vi "WASh controller.vi"(8 "error in (no error)":errorcluster) -> (0 "error out":errorcluster)   [LabVIEW 2015]
doc: "Controller performs all mathematical and logical operations of the application. It is an independent module which communicates with othe modules sending and receiving messaging."
uses:
  type defs/WASH controller states.ctl
  type defs/WASH communication module tasks.ctl
  type defs/WASH step selection buttons.ctl
  type defs/WASH indicators.ctl
  type defs/WASH error levels.ctl
  type defs/WASH simulated database tasks.ctl
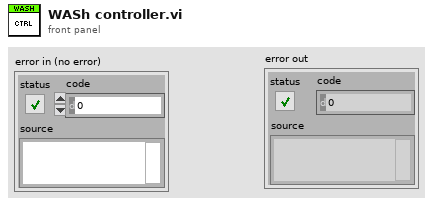
[diagram p1: front panel]
types:
  T1 = typedef "WASH controller states.ctl" = enum16{"initialize", "wait for start", "start", "wait for vehicle position", "wash step execute", "wash step complete", "wash exit", "wash abort"}
  T2 = typedef "WASH error levels.ctl" = enum16{"minor", "wash cycle", "system"}
  T3 = typedef "WASH communication module tasks.ctl" = enum16{"init", "enable controls", "update wash indicators", "update wash entry", "update vehicle out of pos", "update timing", "set step buttons values", "set start button value", "set vehicle position entry", "wait for input", "close"}
  T4 = typedef "WASH simulated database tasks.ctl" = enum16{"init", "read", "insert record", "update record", "query timing", "close"}
  T5 = typedef "WASH indicators.ctl" = cluster{"Under body wash":bool, "bug remover":bool, "Pre-soak":bool, "High pressure wash":bool, "Low pressure wax":bool, "Spot free rinse":bool, "Tire shine foam":bool, "Air dry":bool}
  T6 = typedef "WASH step selection buttons.ctl" = cluster{"Under body wash":bool, "Bug remover":bool, "Pre-soak":bool, "High pressure wash":bool, "Low pressure wax":bool, "Spot free rinse":bool, "Tire shine foam":bool, "Air dry":bool}
  T7 = enum8{"Enabled", "Disabled", "Disabled and Grayed Out"}
  T8 = typedef "WASH UI to CTRL commands.ctl" = enum16{"start button pushed", "vehicle position changed"}
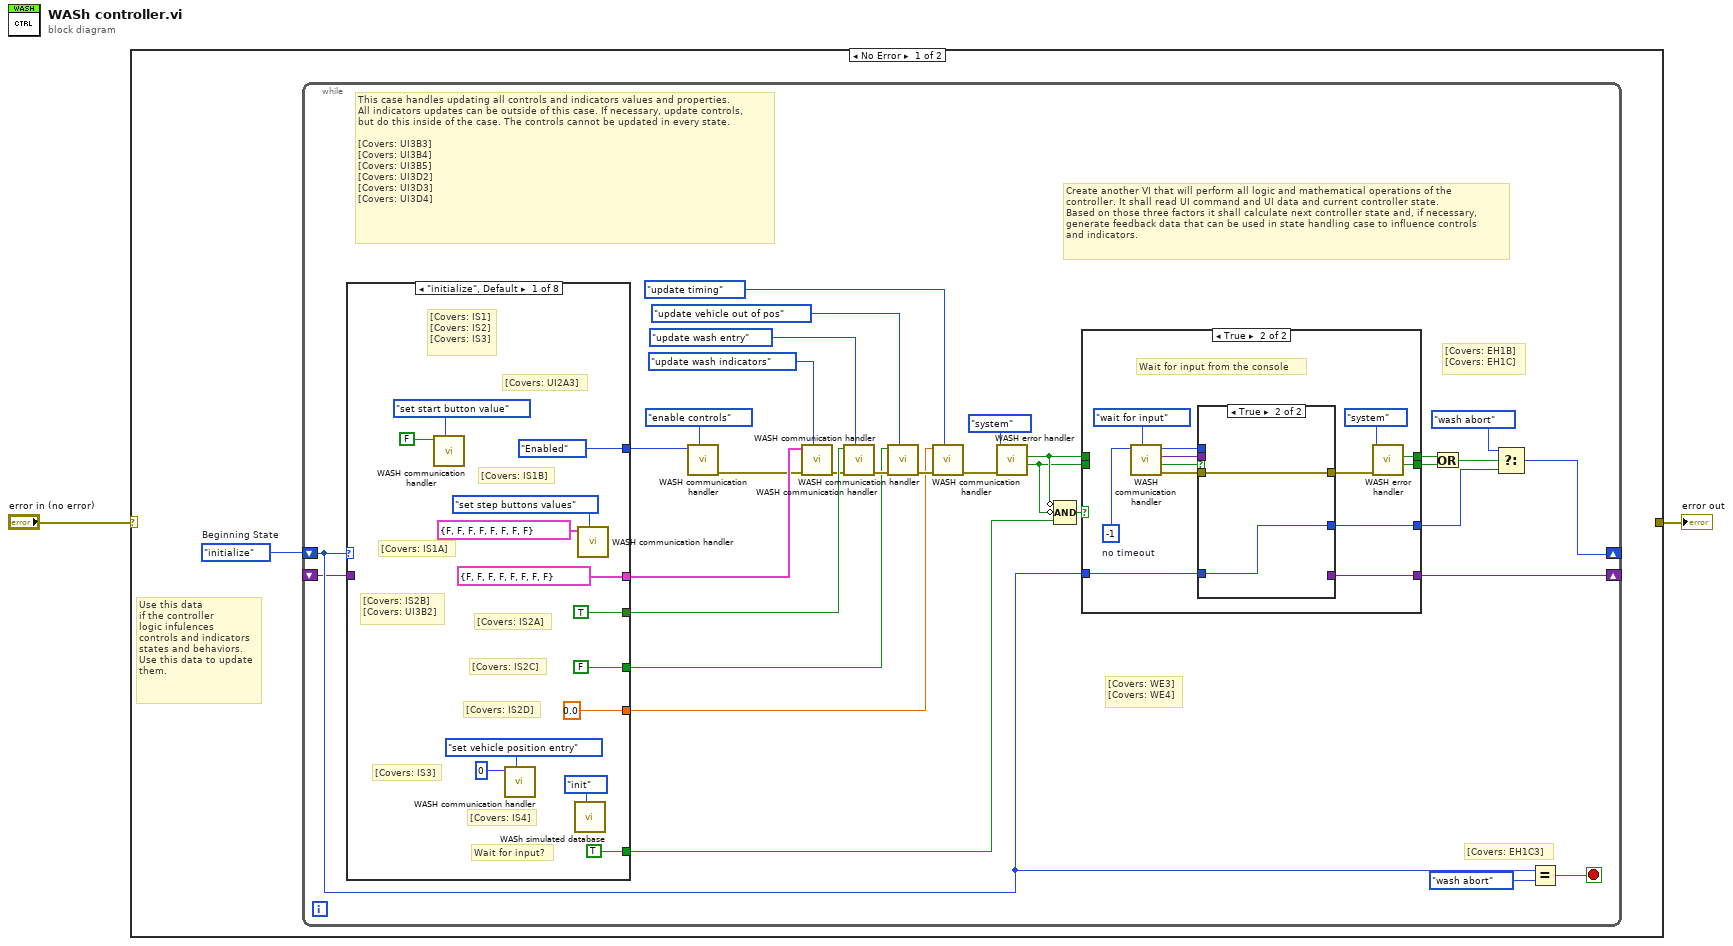
[diagram p0: block diagram]
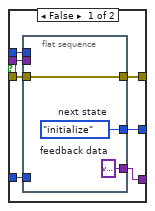
[diagram p3: hidden frame]
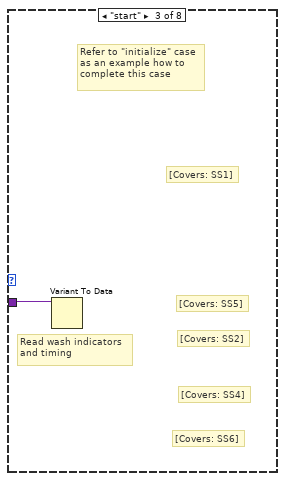
[diagram p5: hidden frame]
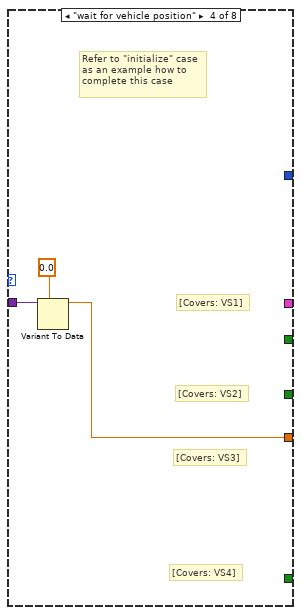
[diagram p6: hidden frame]
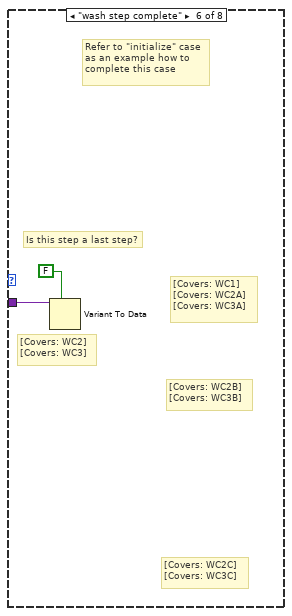
[diagram p8: hidden frame]
diagram:
  n1 = case shown="No Error" "error in (no error)" {
    selector: "error in (no error)" -> [_ w82]
    tunnel: [_ w82] -> w1
    frame No Error {
      w3 = WASH_controller_states."initialize"  # Beginning State
      # "Use this data\nif the controller\nlogic infulences\ncontrols and indicators\nstates and behaviors.\nUse this data to update\nthem."
      n2 = while {
        shift-right: [w9] -> _
        shift-left: w3 -> [w8]
        shift-right: [w4] -> _
        shift-left: _ -> [w5]
        stop <- w7 stop-if-true
        # "[Covers: WE3]\n[Covers: WE4]"
        # "Create another VI that will perform all logic and mathematical operations of the\ncontroller. It shall read UI command and UI data and current controller state.\nBased on those three factors it shall calculate next controller state and, if necessary,\ngenerate feedback data that can be used in state handling case to influence controls\nand indicators."
        # "[Covers: EH1C3]"
        # "[Covers: EH1B]\n[Covers: EH1C]"
        # "This case handles updating all controls and indicators values and properties.\nAll indicators updates can be outside of this case. If necessary, update controls,\nbut do this inside of the case. The controls cannot be updated in every state.\n\n[Covers: UI3B3]\n[Covers: UI3B4]\n[Covers: UI3B5]\n[Covers: UI3D2]\n[Covers: UI3D3]\n[Covers: UI3D4]"
        n3 = case shown="\"initialize\", Default" w8 {
          tunnel: [T7."Enabled" ("Disabled") _ _ _ _ _ _ _] -> w33
          tunnel: [T5 {"Under body wash"=FALSE, "bug remover"=FALSE, "Pre-soak"=FALSE, "High pressure wash"=FALSE, "Low pressure wax"=FALSE, "Spot free rinse"=FALSE, "Tire shine foam"=FALSE, "Air dry"=FALSE} ("wash indicators") _ _ _ _ _ _ _] -> w31
          tunnel: [TRUE _ _ _ _ _ _ _] -> w29
          tunnel: [FALSE _ _ _ _ _ _ _] -> w25
          tunnel: [0.0 _ _ w77 _ _ _ _] -> w21
          tunnel: [TRUE _ _ _ _ _ _ _] -> w15
          tunnel: w5 -> [_ _ w76 w79 _ w81 _ _]
          frame "initialize", Default {
            # "[Covers: UI2A3]"
            # "Wait for input?"
            # "[Covers: IS4]"
            # "[Covers: IS3]"
            # "[Covers: IS2D]"
            # "[Covers: IS2C]"
            # "[Covers: IS1]\n[Covers: IS2]\n[Covers: IS3]"
            # "[Covers: IS2A]"
            # "[Covers: IS2B]\n[Covers: UI3B2]"
            # "[Covers: IS1B]"
            # "[Covers: IS1A]"
            n4 = call "WASH communication handler.vi"("task"=WASH_communication_module_tasks."set start button value", "parameters"=FALSE) -> ()  [unwired: 6 in, 4 out]
            n5 = call "WASH communication handler.vi"("task"=WASH_communication_module_tasks."set vehicle position entry", "parameters"=0) -> ()  [unwired: 6 in, 4 out]
            n6 = call "WASh simulated database.vi"("task"=WASH_simulated_database_tasks."init") -> ()  [unwired: 8 in, 3 out]
            n7 = call "WASH communication handler.vi"("task"=WASH_communication_module_tasks."set step buttons values", "parameters"=T6 {"Under body wash"=FALSE, "Bug remover"=FALSE, "Pre-soak"=FALSE, "High pressure wash"=FALSE, "Low pressure wax"=FALSE, "Spot free rinse"=FALSE, "Tire shine foam"=FALSE, "Air dry"=FALSE} ("Wash step selection")) -> ()  [unwired: 6 in, 4 out]
          }
          frame "wait for start" {
            # "[Covers: WS3]"
            # "[Covers: WS2]"
            # "[Covers: WS1]"
            # "Refer to \"initialize\" case\nas an example how to\ncomplete this case"
          }
          frame "start" {
            # "Read wash indicators\nand timing"
            # "[Covers: SS6]"
            # "[Covers: SS5]"
            # "[Covers: SS4]"
            # "[Covers: SS2]"
            # "Refer to \"initialize\" case\nas an example how to\ncomplete this case"
            # "[Covers: SS1]"
            n8 = Variant To Data(Variant=w76) -> ()  [unwired: 2 in, 2 out]
          }
          frame "wait for vehicle position" {
            # "[Covers: VS4]"
            # "[Covers: VS3]"
            # "[Covers: VS2]"
            # "Refer to \"initialize\" case\nas an example how to\ncomplete this case"
            # "[Covers: VS1]"
            n9 = Variant To Data(type=0.0, Variant=w79) -> (data=w77:dbl)  [unwired: 1 in, 1 out]
          }
          frame "wash step execute" {
            # "[Covers: WX4]"
            # "[Covers: WX3]"
            # "[Covers: WX1]"
            # "[Covers: WX2]"
            # "Refer to \"initialize\" case\nas an example how to\ncomplete this case"
          }
          frame "wash step complete" {
            # "[Covers: WC2C]\n[Covers: WC3C]"
            # "[Covers: WC2B]\n[Covers: WC3B]"
            # "[Covers: WC2]\n[Covers: WC3]"
            # "Is this step a last step?"
            # "Refer to \"initialize\" case\nas an example how to\ncomplete this case"
            # "[Covers: WC1]\n[Covers: WC2A]\n[Covers: WC3A]"
            n10 = Variant To Data(type=FALSE, Variant=w81) -> ()  [unwired: 1 in, 2 out]
          }
          frame "wash exit" {
            # "[Covers: WE2]"
            # "[Covers: WE1]"
            # "Refer to \"initialize\" case\nas an example how to\ncomplete this case"
          }
          frame "wash abort" {
            # "[Covers: TS2]"
            # "[Covers: TS5]"
            # "[Covers: TS4]"
            # "[Covers: TS3]"
            # "[Covers: TS1]"
            # "Refer to \"initialize\" case\nas an example how to\ncomplete this case"
          }
        }
        n11 = call "WASH communication handler.vi"("task"=WASH_communication_module_tasks."enable controls", "parameters"=w33) -> ("error out"=w24:errorcluster)  [unwired: 6 in, 3 out]
        n12 = call "WASH communication handler.vi"("task"=WASH_communication_module_tasks."update wash indicators", "error in (no error)"=w24, "parameters"=w31) -> ("error out"=w28:errorcluster)  [unwired: 5 in, 3 out]
        n13 = call "WASH communication handler.vi"("task"=WASH_communication_module_tasks."update wash entry", "error in (no error)"=w28, "parameters"=w29) -> ("error out"=w27:errorcluster)  [unwired: 5 in, 3 out]
        n14 = call "WASH communication handler.vi"("task"=WASH_communication_module_tasks."update vehicle out of pos", "error in (no error)"=w27, "parameters"=w25) -> ("error out"=w23:errorcluster)  [unwired: 5 in, 3 out]
        n15 = call "WASH communication handler.vi"("task"=WASH_communication_module_tasks."update timing", "error in (no error)"=w23, "parameters"=w21) -> ("error out"=w20:errorcluster)  [unwired: 5 in, 3 out]
        n16 = call "WASH error handler.vi"("error in (no error)"=w20, "error levels"=WASH_error_levels."system") -> ("system error?"=w16:bool, "wash cycle error?"=w17:bool)  [unwired: 7 in, 1 out]
        n17 = Compound Arithmetic op=AND(invert w17, invert w16, w15) -> (w18:bool)
        n18 = case shown="True" w18 {
          tunnel: [w36 w43] -> w12
          tunnel: [w37 w42] -> w10
          tunnel: w17 -> [w37 _]
          tunnel: w16 -> [w36 _]
          tunnel: w8 -> [w35 w40]
          tunnel: [w35 w39] -> w14
          tunnel: [_ w38] -> w4
          frame False {
          }
          frame True {
            w41 = -1  # no timeout
            # "Wait for input from the console"
            n19 = call "WASH communication handler.vi"("task"=WASH_communication_module_tasks."wait for input", "parameters"=w41) -> ("error out"=w48:errorcluster, "timed out?"=w49:bool, "UI data"=w47:variant, "UI command"=w46:T8)  [unwired: 6 in]
            n20 = case shown="True" w49 {
              tunnel: w48 -> [w57 w62]
              tunnel: w47 -> [w54 _]
              tunnel: w46 -> [w53 _]
              tunnel: [w56 w62] -> w45
              tunnel: w40 -> [w55 w61]
              tunnel: [w52 w61] -> w39
              tunnel: [w51 _] -> w38
              frame False {
                n21 = flat-sequence {
                  tunnel: w57 -> [w60]
                  tunnel: [w60] -> w56
                  tunnel: w55 -> [_]
                  tunnel: w54 -> [_]
                  tunnel: w53 -> [_]
                  tunnel: [w59] -> w52
                  tunnel: [w58] -> w51
                  frame #0 {
                    w58 = variant  # feedback data
                    w59 = WASH_controller_states."initialize"  # next state
                  }
                }
              }
              frame True {
              }
            }
            n22 = call "WASH error handler.vi"("error in (no error)"=w45, "error levels"=WASH_error_levels."system") -> ("system error?"=w43:bool, "wash cycle error?"=w42:bool)  [unwired: 7 in, 1 out]
          }
        }
        n23 = Or(x=w10, y=w12) -> (x .or. y?=w11:bool)
        n24 = Select(t=WASH_controller_states."wash abort", s=w11, f=w14) -> (s? t:f=w9:T1)
        n25 = Equal?(x=w8, y=WASH_controller_states."wash abort") -> (x = y?=w7:bool)
      }
    }
    frame Error {
    }
  }
  "error out" <- w1
